vi "Array Size.vi"(11 "Data in":string[][](array[string])) -> (0 "열(I32)":i32, 1 "열(U32)":u32, 2 "행(I32)":i32, 3 "행(U32)":u32)   [LabVIEW 2020]
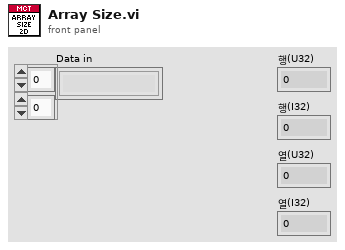
[diagram p1: front panel]
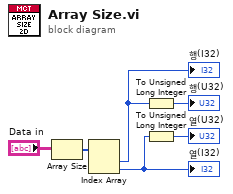
[diagram p0: block diagram]
diagram:
  n1 = Array Size(array="Data in") -> (size(s)=w5:i32[])
  n2 = Index Array(array=w5) -> (element #1=w2:i32, element #2=w1:i32)  [unwired: 2 in]
  "열(I32)" <- w1
  "행(I32)" <- w2
  n3 = To Unsigned Long Integer(number=w2) -> (unsigned 32bit integer=→"행(U32)":u32)
  n4 = To Unsigned Long Integer(number=w1) -> (unsigned 32bit integer=→"열(U32)":u32)
